vi "FindSettingsVariableName.vi"(6 "Seperator (\"\")":string="Channel 1", 8 "error in (no error)":errorcluster, 10 "variable":string, 11 "variant":variant) -> (0 "error out":errorcluster, 3 "cluster name of variable":string)   [LabVIEW 2011]
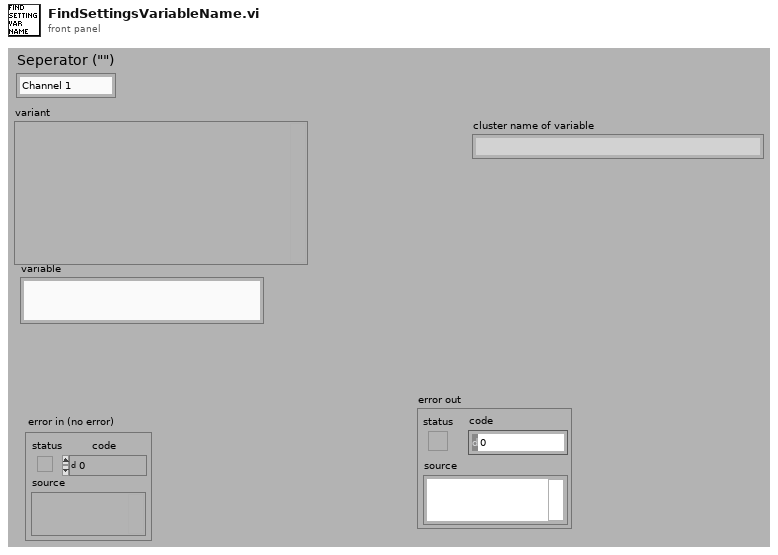
[diagram p1: front panel]
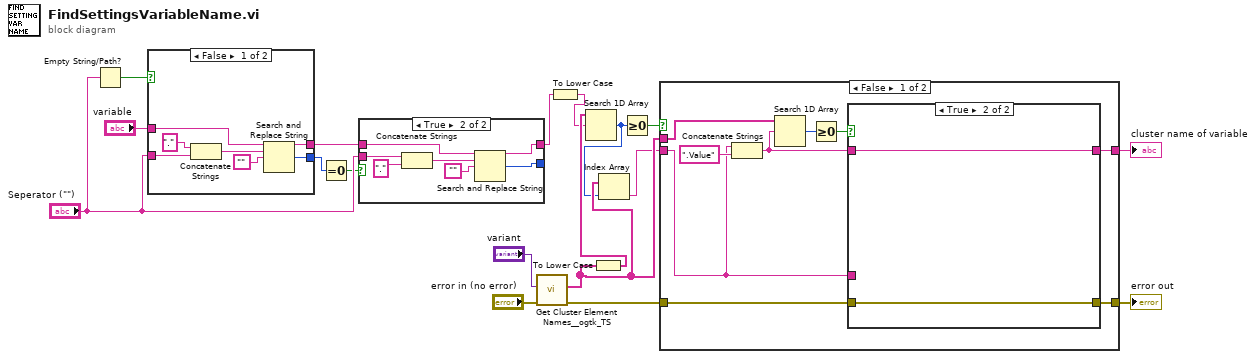
[diagram p0: block diagram]
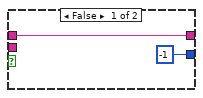
[diagram p2: hidden frame]
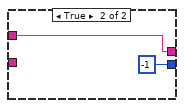
[diagram p3: hidden frame]
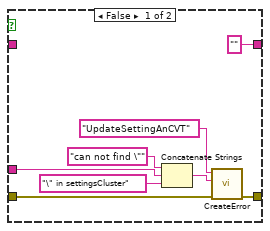
[diagram p4: hidden frame]
diagram:
  n1 = Empty String/Path?(string/path="Seperator (\"\")") -> (empty?=w12:bool)
  n2 = case shown="False" w12 {
    tunnel: "variable" -> [w25 w27]
    tunnel: [w23 w27] -> w7
    tunnel: "Seperator (\"\")" -> [w22 _]
    tunnel: [w19 -1 ("number of replacements")] -> w11
    frame False {
      n3 = Concatenate Strings("." ("string"), w22) -> (w20:string)
      n4 = Search and Replace String(input string=w25, search string=w20, replace string="") -> (result string=w23:string, number of replacements=w19:i32)  [unwired: 5 in, 2 out]
    }
    frame True {
    }
  }
  n5 = Equal To 0?(x=w11) -> (x = 0?=w8:bool)
  n6 = case shown="True" w8 {
    tunnel: w7 -> [w29 w36]
    tunnel: [w29 w34] -> w4
    tunnel: "Seperator (\"\")" -> [_ w33]
    tunnel: [-1 ("number of replacements") w31] -> _
    frame False {
    }
    frame True {
      n7 = Concatenate Strings(w33, "." ("string")) -> (w32:string)
      n8 = Search and Replace String(input string=w36, search string=w32, replace string="") -> (result string=w34:string, number of replacements=w31:i32)  [unwired: 5 in, 2 out]
    }
  }
  n9 = call "Get Cluster Element Names__ogtk_TS.vi"("error in (no error)"="error in (no error)", "Variant"="variant") -> ("error out"=w16:errorcluster, "Names (Array)"=w3:string[])  [unwired: 8 in]
  n10 = To Lower Case(string=w4) -> (all lower case string=w5:string)
  n11 = To Lower Case(string=w3) -> (all lower case string=w6:string[])
  n12 = Search 1D Array(1D array=w6, element=w5) -> (index of element=w2:i32)  [unwired: 1 in]
  n13 = Index Array(array=w3, index=w2) -> (element=w1:string)
  n14 = Greater Or Equal To 0?(x=w2) -> (x >= 0?=w14:bool)
  n15 = case shown="False" w14 {
    tunnel: w1 -> [w37 w57]
    tunnel: [w41 w57] -> w18
    tunnel: w3 -> [w43 _]
    tunnel: w16 -> [w39 w56]
    tunnel: [w38 w56] -> w17
    frame False {
      n16 = Concatenate Strings(w37, ".Value" ("string")) -> (w42:string)
      n17 = Search 1D Array(1D array=w43, element=w42) -> (index of element=w44:i32)  [unwired: 1 in]
      n18 = Greater Or Equal To 0?(x=w44) -> (x >= 0?=w40:bool)
      n19 = case shown="True" w40 {
        tunnel: w42 -> [_ w55]
        tunnel: ["" w55] -> w41
        tunnel: w39 -> [w52 w54]
        tunnel: [w51 w54] -> w38
        tunnel: w37 -> [w48 _]
        frame False {
          n20 = Concatenate Strings("can not find \"" ("error message (\"\")"), w48, "\" in settingsCluster" ("string")) -> (w46:string)
          n21 = call "CreateError.vi"("user error in"=w52, "error message (\"\")"=w46, "command"="UpdateSettingAnCVT") -> ("user error  out"=w51:errorcluster)  [unwired: 8 in]
        }
        frame True {
        }
      }
    }
    frame True {
    }
  }
  "error out" <- w17
  "cluster name of variable" <- w18
